vi "ParseDiffXMLtoPlainText.vi"(0 "XML Path":path, 11 "error in":errorcluster) -> (4 "change description":string, 15 "error out":errorcluster)   [LabVIEW 2020, in "VIDiffScreenshots.lvlib"]
uses:
  VIDiffScreenshots.lvlib
  <vilib>/xml/NI_XML.lvlib
  <resource>/objmgr/DOMUserDefRef.rc
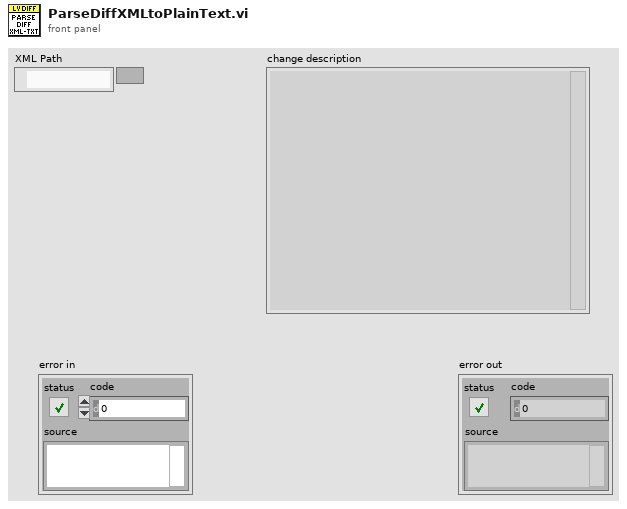
[diagram p1: front panel]
types:
  T1 = cluster{"Value":string, "Value":string, "Value":string, "Value":string}
  T2 = cluster{"Value":string, "Value":string, "Value":string, "Value":string}[]
  T3 = cluster{string, cluster{"Value":string, "Value":string, "Value":string, "Value":string}[]}
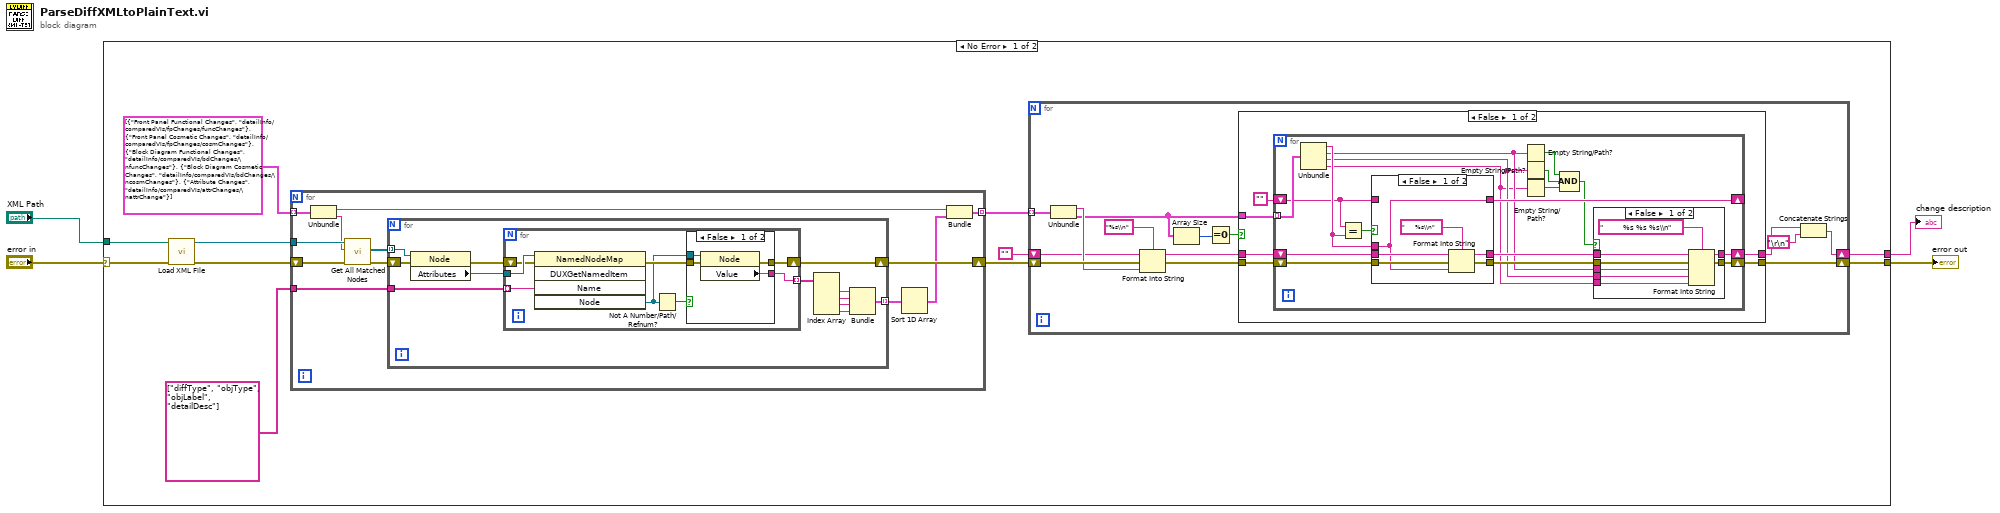
[diagram p0: block diagram]
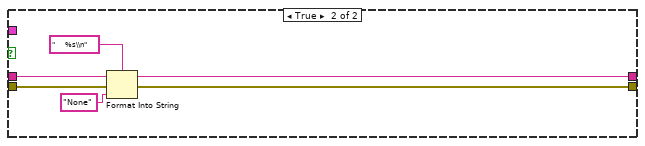
[diagram p4: hidden frame]
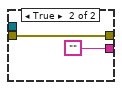
[diagram p5: hidden frame]
diagram:
  n1 = case shown="No Error" "error in" {
    selector: "error in" -> [w15 w117]
    tunnel: "XML Path" -> [w14 _]
    tunnel: [w12 w117] -> w2
    tunnel: [w11 _] -> w1
    frame No Error {
      n2 = call <vilib>:"Load XML File.vi"("path to XML document"=w14, "error in (no error)"=w15) -> ("DOM document out"=w10:refnum<k20>, "error out"=w9:errorcluster)  [unwired: 11 in, 1 out]
      n3 = for {
        tunnel: w10 -> [w90]
        shift-right: [w87] -> w6
        shift-left: w9 -> [w89]
        tunnel: cluster{string, string}[] [{"Front Panel Functional Changes", "detailInfo/comparedVIs/fpChanges/funcChanges"}, {"Front Panel Cosmetic Changes", "detailInfo/comparedVIs/fpChanges/cosmChanges"}, {"Block Diagram Functional Changes", "detailInfo/comparedVIs/bdChanges/\nfuncChanges"}, {"Block Diagram Cosmetic Changes", "detailInfo/comparedVIs/bdChanges/\ncosmChanges"}, {"Attribute Changes", "detailInfo/comparedVIs/attrChanges/\nattrChange"}] -> [w84] mode=indexing
        tunnel: string[] ["diffType", "objType", "objLabel", "detailDesc"] -> [w86]
        tunnel: [w79] -> w8 mode=indexing
        n4 = Unbundle(w84) -> (w80:string, w83:string)
        n5 = call <vilib>:"Get All Matched Nodes.vi"("error in (no error)"=w89, "XPath expression"=w83, "node in"=w90) -> ("error out"=w88:errorcluster, "node result array"=w82:refnum<k20>[])  [unwired: 6 in, 1 out]
        n6 = for {
          shift-right: [w99] -> w87
          shift-left: w88 -> [w100]
          tunnel: w86 -> [w98]
          tunnel: [w92] -> w85 mode=indexing
          tunnel: w82 -> [w91] mode=indexing
          n7 = property class="Node"(reference=w91, error in=w100) -> (error out=w102:errorcluster, "Attributes"=w101:refnum<k20>)  [unwired: 1 out]
          n8 = for {
            tunnel: w101 -> [w110]
            shift-right: [w106] -> w99
            shift-left: w102 -> [w109]
            tunnel: w98 -> [w108] mode=indexing
            tunnel: [w105] -> w97 mode=indexing
            n9 = invoke class="NamedNodeMap" method="DUXGetNamedItem"(reference=w110, error in=w109, "Name"=w108) -> (error out=w107:errorcluster, "Node"=w103:refnum<k20>)  [unwired: 2 in, 3 out]
            n10 = Not A Number/Path/Refnum?(number/path/refnum=w103) -> (NaN/Path/Refnum?=w104:bool)
            n11 = case shown="False" w104 {
              tunnel: w107 -> [w114 w116]
              tunnel: [w113 w116] -> w106
              tunnel: [w112 ""] -> w105
              tunnel: w103 -> [w111 _]
              frame False {
                n12 = property class="Node"(reference=w111, error in=w114) -> (error out=w113:errorcluster, "Value"=w112:string)  [unwired: 1 out]
              }
              frame True {
              }
            }
          }
          n13 = Index Array(array=w97) -> (element #1=w93:string, element #2=w96:string, element #3=w94:string, element #4=w95:string)  [unwired: 4 in]
          n14 = Bundle("Value"=w93, "Value"=w96, "Value"=w94, "Value"=w95) -> (w92:T1)  [unwired: 1 in]
        }
        n15 = Sort 1D Array(array=w85) -> (sorted array=w81:T2)
        n16 = Bundle(w80, w81) -> (w79:T3)  [unwired: 1 in]
      }
      n17 = for {
        tunnel: w8 -> [w29] mode=indexing
        shift-right: [w20] -> w12
        shift-left: w6 -> [w28]
        shift-right: [w17] -> w11
        shift-left: "" -> [w21]
        n18 = Unbundle(w29) -> (w27:string, w19:T2)
        n19 = Format Into String(format string="%s\\n", initial string=w21, error in=w28, w27) -> (resulting string=w22:string, error out=w23:errorcluster)
        n20 = Array Size(array=w19) -> (size(s)=w25:i32)
        n21 = Equal To 0?(x=w25) -> (x = 0?=w24:bool)
        n22 = case shown="False" w24 {
          tunnel: w23 -> [w35 w76]
          tunnel: w22 -> [w34 w75]
          tunnel: [w31 w74] -> w20
          tunnel: [w30 w73] -> w18
          tunnel: w19 -> [w33 _]
          frame False {
            n23 = for {
              shift-right: [w45] -> w31
              shift-left: w35 -> [w51]
              shift-right: [w44] -> w30
              shift-left: w34 -> [w50]
              tunnel: w33 -> [w53] mode=indexing
              shift-right: [w49] -> _
              shift-left: "" -> [w47]
              n24 = Unbundle(w53) -> ("Value"=w48:string, "Value"=w42:string, "Value"=w41:string, "Value"=w40:string)
              n25 = Equal?(x=w47, y=w48) -> (x = y?=w52:bool)
              n26 = case shown="False" w52 {
                tunnel: w51 -> [w68 w72]
                tunnel: w48 -> [w64 _]
                tunnel: w50 -> [w69 w71]
                tunnel: [w66 w72] -> w46
                tunnel: [w65 w71] -> w43
                tunnel: w47 -> [_ w70]
                tunnel: [w64 w70] -> w49
                frame False {
                  n27 = Format Into String(format string="     %s\\n", initial string=w69, error in=w68, w64) -> (resulting string=w65:string, error out=w66:errorcluster)
                }
                frame True {
                }
              }
              n28 = Empty String/Path?(string/path=w42) -> (empty?=w37:bool)
              n29 = Empty String/Path?(string/path=w41) -> (empty?=w38:bool)
              n30 = Empty String/Path?(string/path=w40) -> (empty?=w39:bool)
              n31 = Compound Arithmetic op=AND(w37, w38, w39) -> (w36:bool)
              n32 = case shown="False" w36 {
                tunnel: w46 -> [w61 w62]
                tunnel: [w60 w62] -> w45
                tunnel: [w58 w63] -> w44
                tunnel: w43 -> [w57 w63]
                tunnel: w42 -> [w56 _]
                tunnel: w41 -> [w55 _]
                tunnel: w40 -> [w54 _]
                frame False {
                  n33 = Format Into String(format string="          %s %s %s\\n", initial string=w57, error in=w61, w56, w55, w54) -> (resulting string=w58:string, error out=w60:errorcluster)
                }
                frame True {
                }
              }
            }
          }
          frame True {
            n34 = Format Into String(format string="     %s\\n", initial string=w75, error in=w76, "None" ("input 1")) -> (resulting string=w73:string, error out=w74:errorcluster)
          }
        }
        n35 = Concatenate Strings(w18, "\r\n") -> (w17:string)
      }
    }
    frame Error {
    }
  }
  "error out" <- w2
  "change description" <- w1
